vi "Simple Dataflow Example_MHD.vi"() -> ()   [LabVIEW 2017]
uses:
  C:/Program Files/Princeton Instruments/LightField/PrincetonInstruments.LightFieldAddInSupportServices.dll
  Program Files/Princeton Instruments/LightField/PrincetonInstruments.LightFieldAddInSupportServices.dll
  ProgramData/Documents/Princeton Instruments/LightField/Add-in and Automation SDK/Samples/LabVIEW Automation/lightfield-automation-labview/LightField Automation.lvclass
panel:
  in  "Reset graphs":bool
  out "acquiring data":bool
  in  "Acquire":bool
  in  "Capture":bool=TRUE
  out "Gate End":dbl=870.0
  in  "Gate Width":dbl=10.0 min=0.5 format="%#_13g"
  in  "# Frames":i32=14 min=1
  in  "Gate Start":dbl=740.0 min=1.0 format="%#_13g"
  in  "File":enum32{"File"}(tab)
  in  "Filename":string="Test1"
  out "file path":path=path "E:/LightField/Data/Test/2018-02-05/Test1.tdms"
  in  "base path":path=path "E:/LightField/Data/Test"
  out "Lightfieldpath":path=path "E:/LightField/Data/Test/2018-02-05/LightfieldRaw"
  out "File Size":i64
  in  "Reset capture number":bool
  out "Capture number":i32
  in  "Frame":i32=3
  in  "Tab Control":enum32{"Beam profile timing", "Spectral"}(tab)=enum."Spectral"
  out "Power vs Gate Delay":cluster{dbl[], dbl[]}(graph)={[740.0, 750.0, 760.0, 770.0, 780.0, 790.0, 800.0, 810.0, 820.0, 830.0, 840.0, 850.0, 860.0], [9735.629577636719, 9727.297424316406, 9722.783203125, 9721.853454589844, 9723.992553710938, 9728.69384765625, 9735.276550292969, 9743.003845214844, 9751.08984375, 9758.719848632812, 9764.941833496094, 9768.833984375, 9769.806823730469]}
  out "Gate delay of peak vs time":dbl[](graph)=[860.0]
  out "Capture ROI 1, Frame 1":dbl[][](graph)
  out "Integrated peak vs gate delay":cluster{dbl[], dbl[]}(graph)={[740.0, 750.0, 760.0, 770.0, 780.0, 790.0, 800.0, 810.0, 820.0, 830.0, 840.0, 850.0, 860.0, 870.0, 880.0, 890.0, 900.0, 910.0, 920.0, 930.0, 940.0, 950.0, 960.0, 970.0, 980.0, 990.0, 1000.0, 1010.0, 1020.0, 1030.0, 1040.0, 1050.0, 1060.0, 1070.0, 1080.0, 1090.0, 1100.0, 1110.0, 1120.0, 1130.0, 1140.0, 1150.0, 1160.0, 1170.0, 1180.0, 1190.0, 1200.0, 1210.0, 1220.0, 1230.0, 1240.0, 1250.0, 1260.0, 1270.0, 1280.0, 1290.0, 1300.0, 1310.0, 1320.0, 1330.0, 1340.0, 1350.0, 1360.0, 1370.0, 1380.0, 1390.0, 1400.0, 1410.0, 1420.0, 1430.0, 1440.0, 1450.0, 1460.0, 1470.0, 1480.0, 1490.0, 1500.0, 1510.0, 1520.0, 1530.0], [9735.629577636719, 9727.297424316406, 9722.783203125, 9721.853454589844, 9723.992553710938, 9728.69384765625, 9735.276550292969, 9743.003845214844, 9751.08984375, 9758.719848632812, 9764.941833496094, 9768.833984375, 9769.806823730469, 9767.007446289062, 9759.9833984375, 9747.969177246094, 9735.629577636719, 9727.297424316406, 9722.783203125, 9721.853454589844, 9723.992553710938, 9728.69384765625, 9735.276550292969, 9743.003845214844, 9751.08984375, 9758.719848632812, 9764.941833496094, 9768.833984375, 9769.806823730469, 9767.007446289062, 9759.9833984375, 9747.969177246094, 9735.629577636719, 9727.297424316406, 9722.783203125, 9721.853454589844, 9723.992553710938, 9728.69384765625, 9735.276550292969, 9743.003845214844, 9751.08984375, 9758.719848632812, 9764.941833496094, 9768.833984375, 9769.806823730469, 9767.007446289062, 9759.9833984375, 9747.969177246094, 9735.629577636719, 9727.297424316406, 9722.783203125, 9721.853454589844, 9723.992553710938, 9728.69384765625, 9735.276550292969, 9743.003845214844, 9751.08984375, 9758.719848632812, 9764.941833496094, 9768.833984375, 9769.806823730469, 9767.007446289062, 9759.9833984375, 9747.969177246094, 9735.629577636719, 9727.297424316406, 9722.783203125, 9721.853454589844, 9723.992553710938, 9728.69384765625, 9735.276550292969, 9743.003845214844, 9751.08984375, 9758.719848632812, 9764.941833496094, 9768.833984375, 9769.806823730469, 9767.007446289062, 9759.9833984375, 9747.969177246094]}
  in  "Center WL":dbl=500.0 format="%#_13g"
  in  "WL width":dbl=5.0 format="%#_13g"
  out "Spectra":cluster{dbl[], dbl[]}(graph)={[740.0, 750.0, 760.0, 770.0, 780.0, 790.0, 800.0, 810.0, 820.0, 830.0, 840.0, 850.0, 860.0, 870.0, 880.0, 890.0, 900.0, 910.0, 920.0, 930.0, 940.0, 950.0, 960.0, 970.0, 980.0, 990.0, 1000.0, 1010.0, 1020.0, 1030.0, 1040.0, 1050.0, 1060.0, 1070.0, 1080.0, 1090.0, 1100.0, 1110.0, 1120.0, 1130.0, 1140.0, 1150.0, 1160.0, 1170.0, 1180.0, 1190.0, 1200.0, 1210.0, 1220.0, 1230.0, 1240.0, 1250.0, 1260.0, 1270.0, 1280.0, 1290.0, 1300.0, 1310.0, 1320.0, 1330.0, 1340.0, 1350.0, 1360.0, 1370.0, 1380.0, 1390.0, 1400.0, 1410.0, 1420.0, 1430.0, 1440.0, 1450.0, 1460.0, 1470.0, 1480.0, 1490.0, 1500.0, 1510.0, 1520.0, 1530.0], [9735.629577636719, 9727.297424316406, 9722.783203125, 9721.853454589844, 9723.992553710938, 9728.69384765625, 9735.276550292969, 9743.003845214844, 9751.08984375, 9758.719848632812, 9764.941833496094, 9768.833984375, 9769.806823730469, 9767.007446289062, 9759.9833984375, 9747.969177246094, 9735.629577636719, 9727.297424316406, 9722.783203125, 9721.853454589844, 9723.992553710938, 9728.69384765625, 9735.276550292969, 9743.003845214844, 9751.08984375, 9758.719848632812, 9764.941833496094, 9768.833984375, 9769.806823730469, 9767.007446289062, 9759.9833984375, 9747.969177246094, 9735.629577636719, 9727.297424316406, 9722.783203125, 9721.853454589844, 9723.992553710938, 9728.69384765625, 9735.276550292969, 9743.003845214844, 9751.08984375, 9758.719848632812, 9764.941833496094, 9768.833984375, 9769.806823730469, 9767.007446289062, 9759.9833984375, 9747.969177246094, 9735.629577636719, 9727.297424316406, 9722.783203125, 9721.853454589844, 9723.992553710938, 9728.69384765625, 9735.276550292969, 9743.003845214844, 9751.08984375, 9758.719848632812, 9764.941833496094, 9768.833984375, 9769.806823730469, 9767.007446289062, 9759.9833984375, 9747.969177246094, 9735.629577636719, 9727.297424316406, 9722.783203125, 9721.853454589844, 9723.992553710938, 9728.69384765625, 9735.276550292969, 9743.003845214844, 9751.08984375, 9758.719848632812, 9764.941833496094, 9768.833984375, 9769.806823730469, 9767.007446289062, 9759.9833984375, 9747.969177246094]}
  in  "Aquisition mode":T1(ring)=enum."Spectral Emission Intensity"
  out "Time":dbl=770.0
  in  "Remove first page?":bool=TRUE
  out "TDMS error":errorcluster
  out "TDMS file":refnum<k34>
  in  "stop":bool
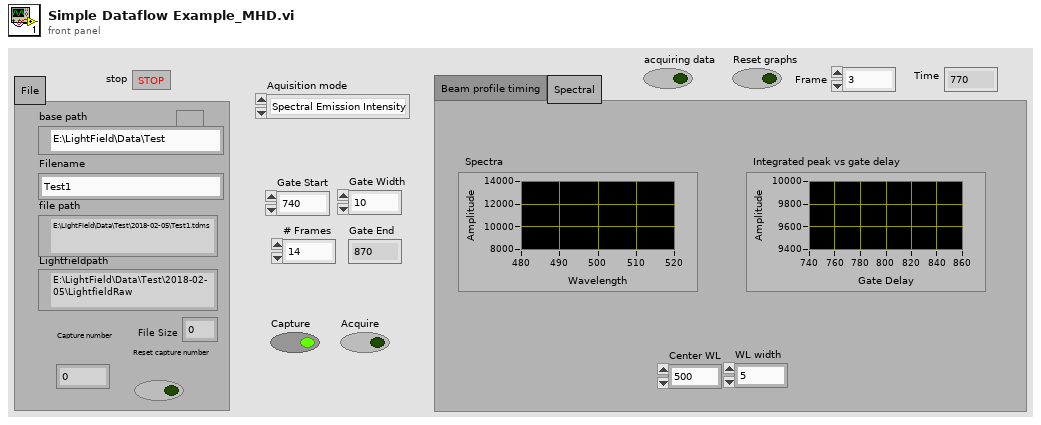
[diagram p1: front panel]
types:
  T1 = enum16{"Beam Profile Power", "Spectral Emission Intensity"}
  T2 = cluster{"Image":dbl[][][], "Frame Size":cluster{"F":i32, "Y":i32, "X":i32}}[]
  T3 = cluster{"Image":dbl[][][], "Frame Size":cluster{"F":i32, "Y":i32, "X":i32}}
  T4 = cluster{"ColumnCalibration":dbl[], "Image":dbl[]}
  T5 = cluster{"Gate Delay Array":dbl[], "Avg Power each frame":dbl[]}
  T6 = enum16{"open", "open or create", "create or replace", "create", "open (read-only)"}
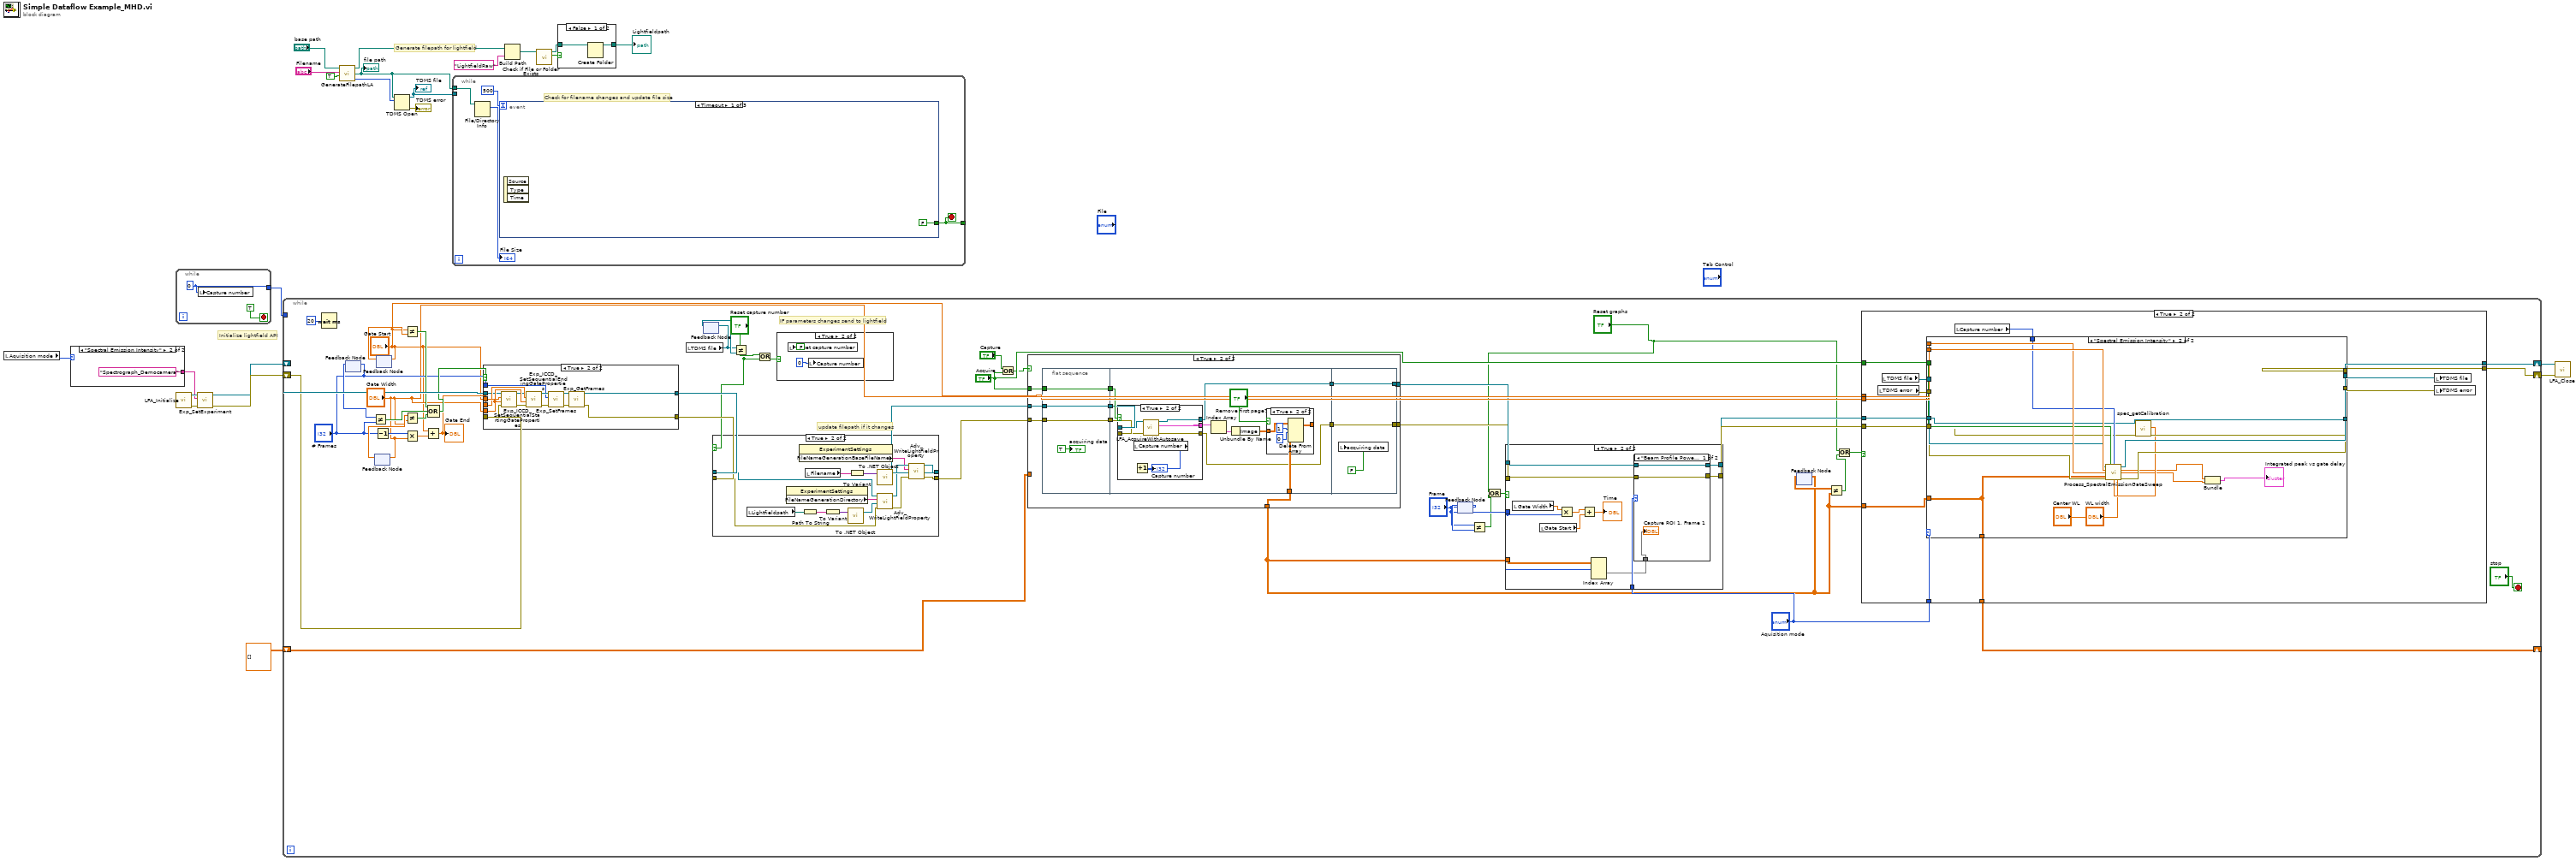
[diagram p0: block diagram]
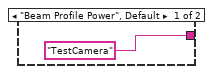
[diagram p2: hidden frame]
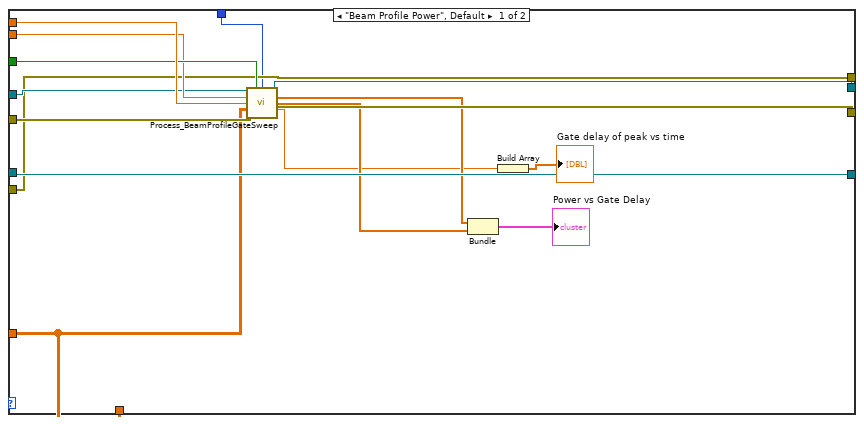
[diagram p4: hidden frame]
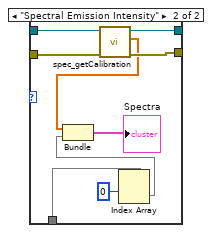
[diagram p6: hidden frame]
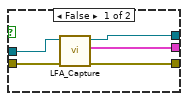
[diagram p9: hidden frame]
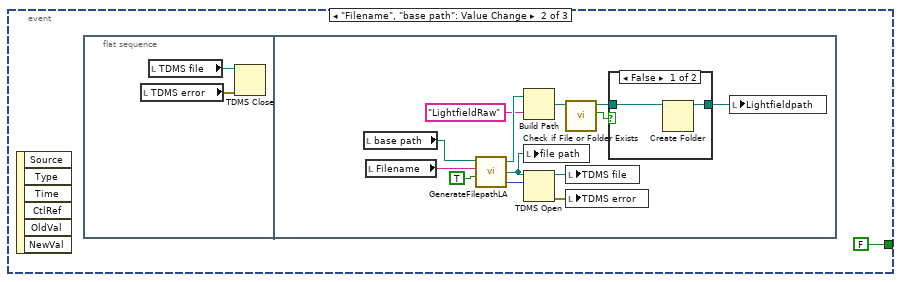
[diagram p14: hidden frame]
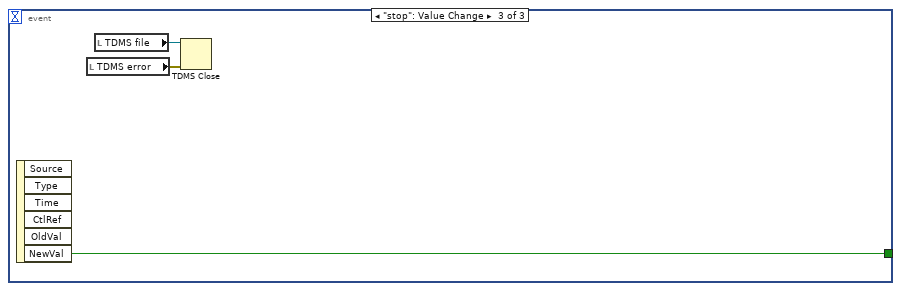
[diagram p16: hidden frame]
diagram:
  # "Initialize lightfield API"
  # "Generate filepath for lightfield"
  n1 = local read "Aquisition mode"() -> (w1:T1)
  n2 = case shown="\"Spectral Emission Intensity\"" w1 {
    tunnel: ["TestCamera" ("ExperimentName") "Spectrograph_Democamera" ("ExperimentName")] -> w12
    frame "Beam Profile Power", Default {
    }
    frame "Spectral Emission Intensity" {
    }
  }
  n3 = while {
    tunnel: [w26] -> w6
    stop <- TRUE stop-if-true
    w26 = 0 ("Capture number")
    n4 = local write "Capture number"(w26) -> ()
  }
  n5 = call "LFA_Initialize.vi"() -> ("error out"=w13:errorcluster, "LightField Automation out"=w14:refnum<class "LightField Automation.lvclass">)  [unwired: 10 in]
  n6 = call "Exp_SetExperiment.vi"("error in (no error)"=w13, "ExperimentName"=w12, "LightField Automation in"=w14) -> ("error out"=w11:errorcluster, "LightField Automation out"=w10:refnum<class "LightField Automation.lvclass">)  [unwired: 7 in]
  n7 = while {
    shift-right: [w73] -> w8
    shift-left: w10 -> [w69]
    shift-right: [w72] -> w9
    shift-left: w11 -> [w68]
    shift-right: [w29] -> _
    shift-left: dbl[][][] [] ("Image") -> [w43]
    tunnel: w6 -> [_]
    stop <- "stop" stop-if-true
    # "update filepath if it changes"
    # "IF parameters changes send to lightfield"
    n8 = Wait (ms)(milliseconds to wait=u32 20) -> ()  [unwired: 1 out]
    n9 = feedback #1() -> (w64:i32)  [unwired: 1 in]
    n10 = feedback-in #1("# Frames") -> ()
    n11 = Not Equal?(x=w64, y="# Frames") -> (x != y?=w65:bool)
    n12 = feedback #2() -> (w63:dbl)  [unwired: 1 in]
    n13 = feedback-in #2("Gate Width") -> ()
    n14 = Decrement(x="# Frames") -> (x-1=w60:i32)
    n15 = feedback #3() -> (w71:dbl)  [unwired: 1 in]
    n16 = feedback-in #3("Gate Start") -> ()
    n17 = Not Equal?(x="Gate Start", y=w71) -> (x != y?=w67:bool)
    n18 = Not Equal?(x=w63, y="Gate Width") -> (x != y?=w66:bool)
    n19 = Multiply(x=w60, y="Gate Width") -> (x*y=w70:dbl)
    n20 = Add(x="Gate Start", y=w70) -> (x+y=w59:dbl)
    "Gate End" <- w59
    n21 = Compound Arithmetic op=OR(w67, w65, w66) -> (w62:bool)
    n22 = case shown="True" w62 {
      tunnel: w69 -> [w220 w225]
      tunnel: w68 -> [w219 w224]
      tunnel: "Gate Start" -> [_ w234]
      tunnel: [w220 w227] -> w54
      tunnel: [w219 w228] -> w53
      tunnel: w59 -> [_ w233]
      tunnel: "Gate Width" -> [_ w226]
      tunnel: "# Frames" -> [_ w221]
      frame False {
      }
      frame True {
        n23 = call "Exp_ICCD_SetSequentialStartingGateProperties.vi"("error in (no error)"=w224, "Sequential Starting Gate Width (ns)"=w226, "Sequential Starting Gate Delay (ns)"=w234, "LightField Automation in"=w225) -> ("error out"=w222:errorcluster, "LightField Automation out"=w223:refnum<class "LightField Automation.lvclass">)  [unwired: 6 in]
        n24 = call "Exp_ICCD_SetSequentialEndingGateProperties.vi"("error in (no error)"=w222, "Sequential Ending Gate Width (ns)"=w226, "Sequential Ending Gate Delay (ns)"=w233, "LightField Automation in"=w223) -> ("error out"=w229:errorcluster, "LightField Automation out"=w230:refnum<class "LightField Automation.lvclass">)  [unwired: 6 in]
        n25 = call "Exp_SetFrames.vi"("error in (no error)"=w229, "Number of Frames"=w221, "LightField Automation in"=w230) -> ("error out"=w232:errorcluster, "LightField Automation out"=w231:refnum<class "LightField Automation.lvclass">)  [unwired: 7 in]
        n26 = call "Exp_GetFrames.vi"("error in (no error)"=w232, "LightField Automation in"=w231) -> ("error out"=w228:errorcluster, "LightField Automation out"=w227:refnum<class "LightField Automation.lvclass">)  [unwired: 7 in, 1 out]
      }
    }
    n27 = local read "TDMS file"() -> (w51:refnum<k34>)
    n28 = feedback #4() -> (w52:refnum<k34>)  [unwired: 1 in]
    n29 = feedback-in #4(w51) -> ()
    n30 = Not Equal?(x=w51, y=w52) -> (x != y?=w48:bool)
    n31 = case shown="True" w48 {
      tunnel: w54 -> [w203 w218]
      tunnel: w53 -> [w202 w217]
      tunnel: [w203 w209] -> w46
      tunnel: [w202 w208] -> w45
      frame False {
      }
      frame True {
        n32 = local read "Lightfieldpath"() -> (w212:path)
        n33 = property class="ExperimentSettings"() -> ("FileNameGenerationDirectory"=w214:string)  [unwired: 2 in, 2 out]
        n34 = property class="ExperimentSettings"() -> ("FileNameGenerationBaseFileName"=w204:string)  [unwired: 2 in, 2 out]
        n35 = Path To String(path=w212) -> (string=w216:string)
        n36 = local read "Filename"() -> (w210:string)
        n37 = To Variant(anything=w216) -> (Variant=w215:variant)
        n38 = call <vilib>:"To .NET Object.vi"("anything"=w215) -> (".NET object"=w213:refnum<k24>)  [unwired: 1 in, 1 out]
        n39 = To Variant(anything=w210) -> (Variant=w211:variant)
        n40 = call <vilib>:"To .NET Object.vi"("anything"=w211) -> (".NET object"=w205:refnum<k24>)  [unwired: 1 in, 1 out]
        n41 = call "Adv_WriteLightFieldProperty.vi"("error in (no error)"=w217, "value"=w213, "setting"=w214, "LightField Automation in"=w218) -> ("error out"=w206:errorcluster, "LightField Automation out"=w207:refnum<class "LightField Automation.lvclass">)  [unwired: 6 in]
        n42 = call "Adv_WriteLightFieldProperty.vi"("error in (no error)"=w206, "value"=w205, "setting"=w204, "LightField Automation in"=w207) -> ("error out"=w208:errorcluster, "LightField Automation out"=w209:refnum<class "LightField Automation.lvclass">)  [unwired: 6 in]
      }
    }
    n43 = Or(x="Reset capture number", y=w48) -> (x .or. y?=w47:bool)
    n44 = case shown="True" w47 {
      frame False {
      }
      frame True {
        n45 = local write "Reset capture number"(FALSE ("Reset")) -> ()
        n46 = local write "Capture number"(0 ("Capture number")) -> ()
      }
    }
    n47 = Or(x="Capture", y="Acquire") -> (x .or. y?=w44:bool)
    n48 = case shown="True" w44 {
      tunnel: "Acquire" -> [_ w167]
      tunnel: w46 -> [w156 w166]
      tunnel: w45 -> [w155 w165]
      tunnel: [w154 w164] -> w34
      tunnel: [w156 w163] -> w40
      tunnel: [w155 w162] -> w39
      tunnel: w43 -> [w154 _]
      frame False {
      }
      frame True {
        n49 = flat-sequence {
          tunnel: w165 -> [w169]
          tunnel: w166 -> [w170]
          tunnel: w167 -> [w171]
          tunnel: [w171] -> w161
          tunnel: [w170] -> w160
          tunnel: [w169] -> w159
          tunnel: [w176] -> w164
          tunnel: w161 -> [w181]
          tunnel: w160 -> [w180]
          tunnel: w159 -> [w179]
          tunnel: [w173] -> w158
          tunnel: [w172] -> w157
          tunnel: [w200] -> w162
          tunnel: [w201] -> w163
          tunnel: w158 -> [w201]
          tunnel: w157 -> [w200]
          frame #0 {
            "acquiring data" <- TRUE ("aquiring data")
          }
          frame #1 {
            n50 = case shown="True" w181 {
              tunnel: [w191 w195] -> w172
              tunnel: [w190 w197] -> w173
              tunnel: [w189 w194] -> w177
              tunnel: w180 -> [w188 w198]
              tunnel: w179 -> [w187 w196]
              frame False {
                n51 = call "LFA_Capture.vi"("error in (no error)"=w187, "LightField Automation in"=w188) -> ("error out"=w191:errorcluster, "Data"=w189:T2, "LightField Automation out"=w190:refnum<class "LightField Automation.lvclass">)  [unwired: 7 in]
              }
              frame True {
                n52 = local read "Capture number"() -> (w192:i32)
                n53 = Increment(x=w192) -> (x+1=→"Capture number":i32)
                n54 = call "LFA_AcquireWithAutosave.vi"("error in (no error)"=w196, "LightField Automation in"=w198) -> ("error out"=w195:errorcluster, "Data"=w194:T2, "LightField Automation out"=w197:refnum<class "LightField Automation.lvclass">)  [unwired: 7 in]
              }
            }
            n55 = Index Array(array=w177) -> (element=w178:T3)  [unwired: 1 in]
            n56 = Unbundle By Name(w178) -> ("Image"=w175:dbl[][][])
            n57 = case shown="True" "Remove first page?" {
              tunnel: [w182 w186] -> w176
              tunnel: w175 -> [w182 w185]
              frame False {
              }
              frame True {
                n58 = Delete From Array(array=w185, length=1, index (dim 0)=0 ("index (page)")) -> (array with subset deleted=w186:dbl[][][])  [unwired: 2 in, 1 out]
              }
            }
          }
          frame #2 {
            n59 = local write "acquiring data"(FALSE ("aquiring data")) -> ()
          }
        }
      }
    }
    n60 = feedback #5() -> (w42:i32)  [unwired: 1 in]
    n61 = feedback-in #5("Frame") -> ()
    n62 = Not Equal?(x="Frame", y=w42) -> (x != y?=w30:bool)
    n63 = Or(x="Reset graphs", y=w30) -> (x .or. y?=w31:bool)
    n64 = case shown="True" w31 {
      tunnel: w34 -> [_ w137]
      tunnel: "Frame" -> [_ w136]
      tunnel: w40 -> [w129 w135]
      tunnel: w39 -> [w128 w134]
      tunnel: [w128 w133] -> w38
      tunnel: [w129 w132] -> w37
      tunnel: "Aquisition mode" -> [_ w131]
      frame False {
      }
      frame True {
        n65 = local read "Gate Width"() -> (w141:dbl)
        n66 = local read "Gate Start"() -> (w139:dbl)
        n67 = Multiply(x=w141, y=w136) -> (x*y=w140:dbl)
        n68 = Add(x=w140, y=w139) -> (x+y=→"Time":dbl)
        n69 = Index Array(array=w137, index (dim 0)=w136) -> (element=w130:dbl[][])  [unwired: 2 in]
        n70 = case shown="\"Beam Profile Power\", Default" w131 {
          tunnel: w135 -> [w144 w153]
          tunnel: w134 -> [w143 w152]
          tunnel: [w143 w151] -> w133
          tunnel: [w144 w150] -> w132
          tunnel: w130 -> [w142 w148]
          frame "Beam Profile Power", Default {
            "Capture ROI 1, Frame 1" <- w142
          }
          frame "Spectral Emission Intensity" {
            n71 = call "spec_getCalibration.vi"("error in (no error)"=w152, "LightField Automation in"=w153) -> ("error out"=w151:errorcluster, "ColumnCalibration"=w146:dbl[], "LightField Automation out"=w150:refnum<class "LightField Automation.lvclass">)  [unwired: 7 in]
            n72 = Index Array(array=w148, index (row)=0) -> (element=w147:dbl[])  [unwired: 1 in]
            n73 = Bundle("ColumnCalibration"=w146, "Image"=w147) -> (→"Spectra":T4)  [unwired: 1 in]
          }
        }
      }
    }
    n74 = feedback #6() -> (w35:dbl[][][])  [unwired: 1 in]
    n75 = feedback-in #6(w34) -> ()
    n76 = Not Equal?(x=w35, y=w34) -> (x != y?=w33:bool)
    n77 = Or(x="Reset graphs", y=w33) -> (x .or. y?=w32:bool)
    n78 = case shown="True" w32 {
      tunnel: [w77 w92] -> w73
      tunnel: [w76 w91] -> w72
      tunnel: "Gate Width" -> [_ w90]
      tunnel: "Acquire" -> [_ w89]
      tunnel: "Gate Start" -> [_ w88]
      tunnel: w38 -> [w76 w82]
      tunnel: w37 -> [w77 w81]
      tunnel: "Aquisition mode" -> [_ w80]
      tunnel: w34 -> [w75 w79]
      tunnel: [w75 w78] -> w29
      frame False {
      }
      frame True {
        n79 = local read "TDMS error"() -> (w85:errorcluster)
        n80 = local read "TDMS file"() -> (w84:refnum<k34>)
        n81 = local read "Capture number"() -> (w83:i32)
        n82 = case shown="\"Spectral Emission Intensity\"" w80 {
          tunnel: w90 -> [w108 w126]
          tunnel: w83 -> [w96 w120]
          tunnel: w89 -> [w107 w121]
          tunnel: w79 -> [w93 w109]
          tunnel: w88 -> [w106 w127]
          tunnel: [w105 w122] -> w87
          tunnel: [w104 w124] -> w86
          tunnel: w85 -> [w103 w123]
          tunnel: w84 -> [w102 w125]
          tunnel: w81 -> [w101 w119]
          tunnel: w82 -> [w100 w118]
          tunnel: [w101 w117] -> w92
          tunnel: [w100 w116] -> w91
          tunnel: [w93 w109] -> w78
          frame "Beam Profile Power", Default {
            n83 = call "Process_BeamProfileGateSweep.vi"("Refnum in"=w102, "Acquire"=w107, "Capture number"=w96, "Gate Start"=w106, "Gate Width"=w108, "Image"=w93, "error in (no error)"=w103) -> ("Refnum out"=w104:refnum<k34>, "Gate Delay Array"=w99:dbl[], "Avg Power each frame"=w98:dbl[], "Gate Delay of peak intensity"=w95:dbl, "error out"=w105:errorcluster)  [unwired: 4 in]
            n84 = Bundle("Gate Delay Array"=w99, "Avg Power each frame"=w98) -> (→"Power vs Gate Delay":T5)  [unwired: 1 in]
            n85 = Build Array(w95) -> (→"Gate delay of peak vs time":dbl[])
          }
          frame "Spectral Emission Intensity" {
            n86 = call "spec_getCalibration.vi"("error in (no error)"=w118, "LightField Automation in"=w119) -> ("error out"=w116:errorcluster, "ColumnCalibration"=w115:dbl[], "LightField Automation out"=w117:refnum<class "LightField Automation.lvclass">)  [unwired: 7 in]
            n87 = call "Process_SpectralEmissionGateSweep.vi"("Refnum in"=w125, "Acquire"=w121, "Capture number"=w120, "Center WL"="Center WL", "Gate Start"=w127, "Gate Width"=w126, "Image"=w109, "error in (no error)"=w123, "ColumnCalibration"=w115, "WL width"="WL width") -> ("Refnum out"=w124:refnum<k34>, "Gate Delay Array"=w112:dbl[], "Avg Power each frame"=w111:dbl[], "error out"=w122:errorcluster)  [unwired: 1 in, 1 out]
            n88 = Bundle("Gate Delay Array"=w112, "Avg Power each frame"=w111) -> (→"Integrated peak vs gate delay":T5)  [unwired: 1 in]
          }
        }
        n89 = local write "TDMS file"(w86) -> ()
        n90 = local write "TDMS error"(w87) -> ()
      }
    }
  }
  n91 = call "GenerateFilepathLA.vi"("Auto Date folder"=TRUE, "Filename"="Filename", "base path"="base path") -> ("operation (0:open)"=w19:T6, "file path"=w18:path, "Folder Path"=w16:path)  [unwired: 1 in]
  "file path" <- w18
  n92 = TDMS Open(10:w19, 11:w18) -> (0:→"TDMS error":errorcluster, 3:w17:refnum<k34>)  [unwired: 5 in]
  "TDMS file" <- w17
  n93 = while {
    tunnel: [w237] -> _
    tunnel: w18 -> [w238]
    tunnel: w17 -> [_]
    stop <- w237 stop-if-true
    # "Check for filename changes and update file size"
    n94 = File/Directory Info(path=w238) -> (size=→"File Size":i64)  [unwired: 1 in, 6 out]
    n95 = event shown="[0] Timeout" {
      selector: _ -> [_ _ _]
      dyn-events: _ -> [_ _ _]
      timeout: 500 -> [_ _ _]
      tunnel: [FALSE ("NewVal") FALSE ("NewVal") w263] -> w237
      event Timeout {
        n96 = event-data() -> ()  [unwired: 1 in, 3 out]
      }
      event "Filename", "base path": Value Change {
        n97 = event-data() -> ()  [unwired: 1 in, 6 out]
        n98 = flat-sequence {
          frame #0 {
            n99 = local read "TDMS error"() -> (w244:errorcluster)
            n100 = local read "TDMS file"() -> (w243:refnum<k34>)
            n101 = TDMS Close(8:w244, 11:w243) -> ()  [unwired: 2 out]
          }
          frame #1 {
            n102 = local read "base path"() -> (w257:path)
            n103 = local read "Filename"() -> (w251:string)
            n104 = call "GenerateFilepathLA.vi"("Auto Date folder"=TRUE, "Filename"=w251, "base path"=w257) -> ("operation (0:open)"=w254:T6, "file path"=w256:path, "Folder Path"=w250:path)  [unwired: 1 in]
            n105 = Build Path(base path=w250, name or relative path="LightfieldRaw") -> (appended path=w248:path)
            n106 = local write "file path"(w256) -> ()
            n107 = TDMS Open(10:w254, 11:w256) -> (0:w252:errorcluster, 3:w253:refnum<k34>)  [unwired: 5 in]
            n108 = call <vilib>:"Check if File or Folder Exists.vi"("path"=w248) -> ("file or folder exists?"=w247:bool, "dup path"=w246:path)  [unwired: 8 in, 1 out]
            n109 = local write "TDMS file"(w253) -> ()
            n110 = local write "TDMS error"(w252) -> ()
            n111 = case shown="False" w247 {
              tunnel: w246 -> [w259 w260]
              tunnel: [w258 w260] -> w245
              frame False {
                n112 = Create Folder(path (use dialog)=w259) -> (created path=w258:path)  [unwired: 2 in, 2 out]
              }
              frame True {
              }
            }
            n113 = local write "Lightfieldpath"(w245) -> ()
          }
        }
      }
      event "stop": Value Change {
        n114 = event-data() -> ("NewVal"=w263:bool)  [unwired: 1 in, 5 out]
        n115 = local read "TDMS error"() -> (w262:errorcluster)
        n116 = local read "TDMS file"() -> (w261:refnum<k34>)
        n117 = TDMS Close(8:w262, 11:w261) -> ()  [unwired: 2 out]
      }
    }
  }
  n118 = Build Path(base path=w16, name or relative path="LightfieldRaw") -> (appended path=w2:path)
  n119 = call <vilib>:"Check if File or Folder Exists.vi"("path"=w2) -> ("file or folder exists?"=w4:bool, "dup path"=w5:path)  [unwired: 8 in, 1 out]
  n120 = case shown="False" w4 {
    tunnel: w5 -> [w265 w266]
    tunnel: [w264 w266] -> w3
    frame False {
      n121 = Create Folder(path (use dialog)=w265) -> (created path=w264:path)  [unwired: 2 in, 2 out]
    }
    frame True {
    }
  }
  "Lightfieldpath" <- w3
  n122 = call "LFA_Close.vi"("error in (no error)"=w9, "LightField Automation in"=w8) -> ()  [unwired: 8 in, 2 out]
